vi "Rename Edges.vi"(0 "Display State In":T1, 5 "Old Name":string, 7 "New Name":string, 9 "Container State":T5, 11 "error in (no error)":errorcluster) -> (4 "Display State Out":T1, 15 "error out":errorcluster)   [LabVIEW 2015, in "FSM Editor.xctl"]
uses:
  FSM Editor.xctl
  <vilib>/_xctls/Container State.ctl
  State.vi
  Classes/FSM.Port/FSM.Port.lvclass
  <vilib>/Utility/miscctls.llb/LVPoint32TypeDef.ctl
  Drag Mode.ctl
  Events.ctl
  NodeAdded.ctl
  NodeSelected.ctl
  EdgeEventData.ctl
  <vilib>/_xctls/XControlSupport.lvlib
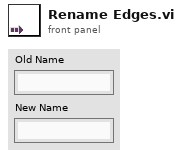
[diagram p1: front panel]
types:
  T1 = typedef "FSM Editor.xctl/State.vi" = cluster{"snap":bool, "default name":string, "dragStartPoint":T2, "dragMode":T3, "gridsize":dbl, "selectRect":cluster{"left":i16, "top":i16, "right":i16, "bottom":i16}, "events":string[], "cs+/cs-":bool, "insertEdgeAt":string, "insertingEdge":bool, "activePort":refnum<class "FSM.Port.lvclass">, "sourcePort":refnum<class "FSM.Port.lvclass">, "insertionEnd":cluster{"x":i16, "y":i16}, "insertEdgeSpec":string, "nodeIndex":i32, "Events":T4, "action":string}
  T2 = typedef "LVPoint32TypeDef.ctl" = cluster{"Horizontal":i32, "Vertical":i32}
  T3 = typedef "Drag Mode.ctl" = enum16{"Off", "NodePending", "Nodes", "Pan", "Select", "EdgeInsertion", "EdgePoint", "EdgeLabel"}
  T4 = typedef "FSM Editor.xctl/Events.ctl" = cluster{"NodeAdded":refnum<user-event>, "NodeSelected":refnum<user-event>, "EdgeAdded":refnum<user-event>, "EdgeDeleted":refnum<user-event>, "EdgeSelected":refnum<user-event>}
  T5 = typedef "XControlSupport.lvlib/Container State.ctl" = cluster{"Indicator?":bool, "Run Mode?":bool, " Refnum":refnum<vi>}
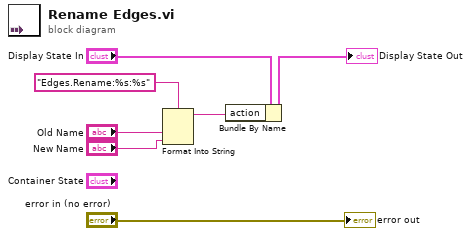
[diagram p0: block diagram]
diagram:
  n1 = Format Into String(format string="Edges.Rename:%s:%s", "Old Name", "New Name") -> (resulting string=w3:string)  [unwired: 2 in, 1 out]
  n2 = Bundle By Name(cluster="Display State In", "action"=w3) -> (→"Display State Out":T1)
  "error out" <- "error in (no error)"
